vi "FTW-CodeGen-GenerateCode.vi"(0 "State In":T2, 5 "XRef":refnum<vi>, 7 "Terms":T1(array[cluster]), 9 "Diagram":refnum<vi>) -> (4 "State Out":T2, 6 "Reply":string[](array[string]), 8 "Generated Code?":bool)   [LabVIEW 2014, in "FTW-Sync-Synchronizer.xnode"]
uses:
  FTW-Sync-Synchronizer.xnode
  FTW-CodeGen-State.ctl
  codegen/FTW-CodeGen-XNodeReplyType.ctl
  FTW-CodeGen-Prototype.vi
panel:
  # "Inputs"
  # "Outputs"
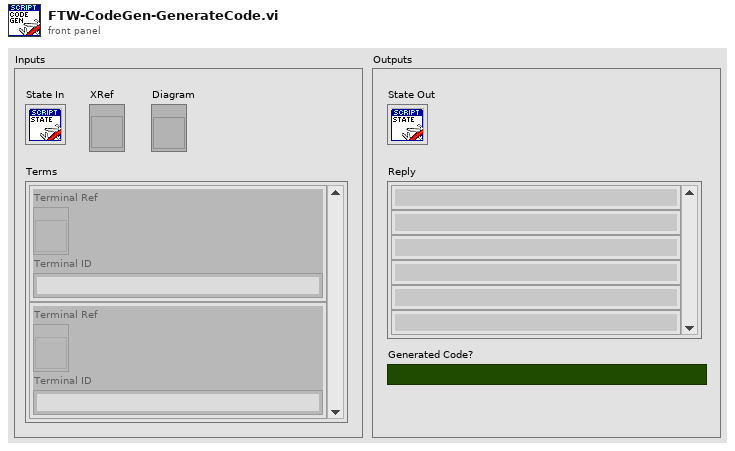
[diagram p1: front panel]
types:
  T1 = cluster{"Terminal Ref":refnum<vi>, "Terminal ID":string}[]
  T2 = typedef "FTW-Sync-Synchronizer.xnode/FTW-CodeGen-State.ctl" = cluster{"InputTerminals":cluster{"Wired?":bool, "ID":string, "DataName":string, "DataColor":u32, "Type":variant}[], "EnableTiming?":bool}
  T3 = typedef "FTW-CodeGen-XNodeReplyType.ctl" = enum16{"UpdateState", "AdaptToInputs", "AdaptAndAugment", "CosmeticUpdate", "NoReply"}
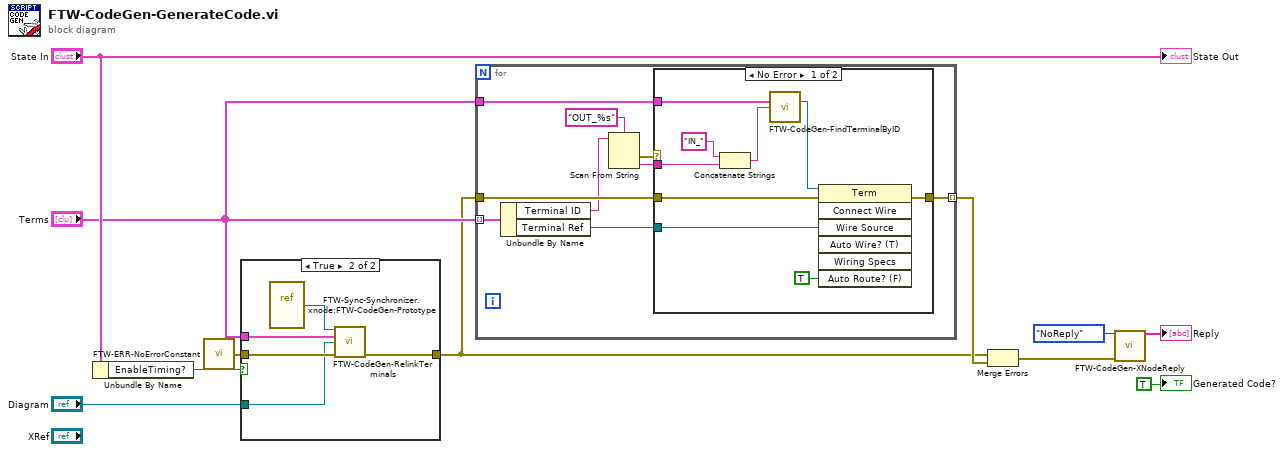
[diagram p0: block diagram]
diagram:
  n1 = Unbundle By Name("State In") -> ("EnableTiming?"=w3:bool)
  n2 = call "FTW-ERR-NoErrorConstant.vi"() -> ("no error"=w5:errorcluster)
  n3 = case shown="True" w3 {
    tunnel: "Terms" -> [_ w17]
    tunnel: w5 -> [w12 w16]
    tunnel: [w12 w13] -> w4
    tunnel: "Diagram" -> [_ w15]
    frame False {
    }
    frame True {
      n4 = vi-ref "FTW-Sync-Synchronizer.xnode:FTW-CodeGen-Prototype.vi"() -> (w14:refnum<vi>)
      n5 = call "FTW-CodeGen-RelinkTerminals.vi"("PrototypeVI"=w14, "Terms"=w17, "Diagram"=w15, "error in"=w16) -> ("error out"=w13:errorcluster)  [unwired: 11 in]
    }
  }
  n6 = for {
    tunnel: "Terms" -> [w26] mode=indexing
    tunnel: [w21] -> w7 mode=indexing
    tunnel: w4 -> [w20]
    tunnel: "Terms" -> [w19]
    n7 = Unbundle By Name(w26) -> ("Terminal ID"=w18:string, "Terminal Ref"=w22:refnum<vi>)
    n8 = Scan From String(format string="OUT_%s", input string=w18) -> (error out=w24:errorcluster, output 1=w23:string)  [unwired: 3 in, 2 out]
    n9 = case shown="No Error" w24 {
      tunnel: w23 -> [w34 _]
      tunnel: w22 -> [w27 _]
      tunnel: [w33 w36] -> w21
      tunnel: w20 -> [w29 w36]
      tunnel: w19 -> [w31 _]
      frame No Error {
        n10 = Concatenate Strings("IN_" ("string"), w34) -> (w32:string)
        n11 = call "FTW-CodeGen-FindTerminalByID.vi"("Terms"=w31, "Terminal ID"=w32) -> ("Terminal Ref"=w30:refnum<vi>)  [unwired: 12 in, 1 out]
        n12 = invoke class="Term" method="Connect Wire"(reference=w30, error in=w29, "Wire Source"=w27, "Auto Route? (F)"=TRUE) -> (error out=w33:errorcluster)  [unwired: 3 in, 6 out]
      }
      frame Error {
      }
    }
  }
  n13 = Merge Errors(w4, w7) -> (w1:errorcluster)
  n14 = call "FTW-CodeGen-XNodeReply.vi"("XNode Reply Type"=FTW-CodeGen-XNodeReplyType."NoReply", "error in"=w1) -> ("Reply"=→"Reply":string[])  [unwired: 13 in]
  "State Out" <- "State In"
  "Generated Code?" <- TRUE ("Generated Code?")
